vi "MOVE BIAS (M).vi"(0 "SweepQ In":refnum<queue>, 1 "x":dbl, 2 "return value":cluster{"x":dbl, "y":dbl}, 5 "ScanQ in":refnum<queue>, 7 "Boolean":bool, 11 "error in (no error)":errorcluster, 12 "y":dbl, 13 "Bias in":T1 {"Final Y (m)" format="%.3p"; "Final X (m)" format="%.3p"}) -> (3 "X (m)":sgl, 4 "SweepQ Out":refnum<queue>, 6 "ScanQ out":refnum<queue>, 14 "Y (m)":sgl, 15 "error out":errorcluster)   [LabVIEW 2025]
uses:
  STM-Auto-Project/QMH CTLS/Scan_Params (QMH).ctl
  LabVIEW VI's/Instrument VI's/Instrument Controls/Magnet Array.ctl
  Magnetic Drift Correction/Bias Cont QMH.ctl
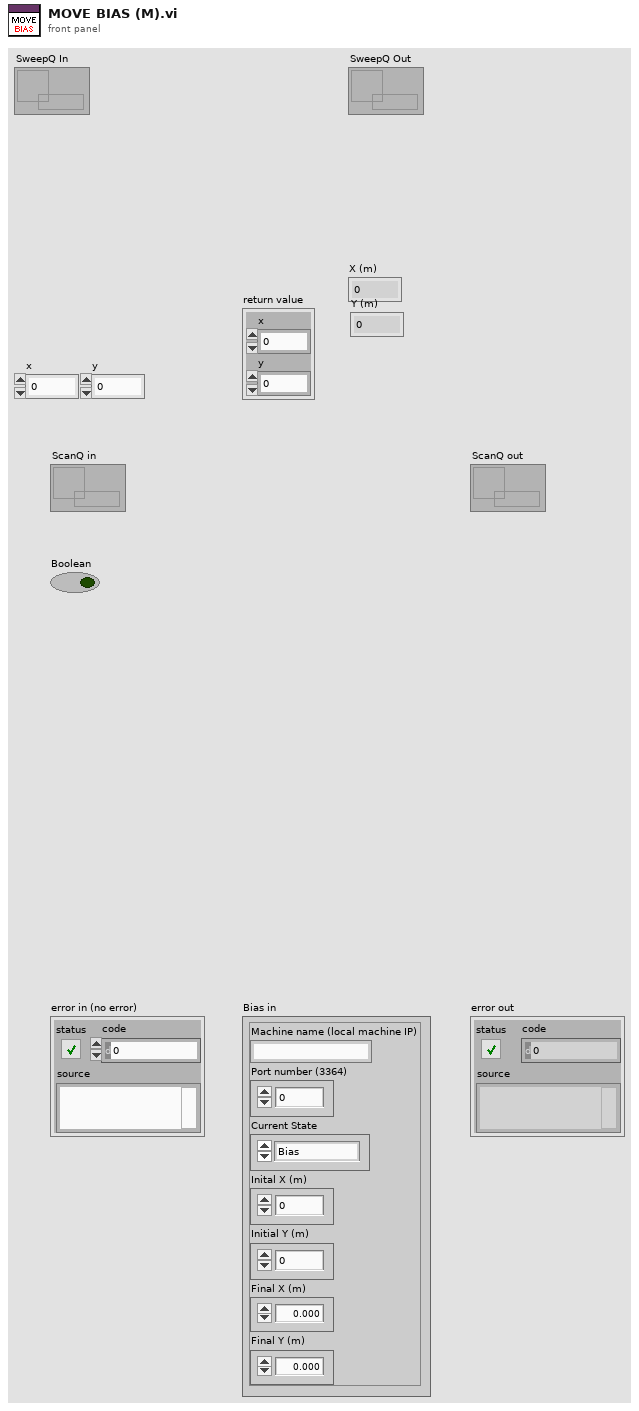
[diagram p1: front panel]
types:
  T1 = typedef "Bias Cont QMH.ctl" = cluster{"Machine name (local machine IP)":string, "Port number (3364)":u32, "Current State":enum16{"Bias", "Stop"}, "Inital X (m)":dbl, "Initial Y (m)":dbl, "Final X (m)":sgl, "Final Y (m)":sgl}
  T2 = enum16{"SET FIELD", "SWEEP IDLE", "NEXT FIELD", "SWEEP DONE"}
  T3 = typedef "Magnet Array.ctl" = cluster{"Sweep States":enum16{"SET FIELD", "SWEEP IDLE", "NEXT FIELD", "SWEEP DONE"}, "VISA Connection":refnum<visa-resource-name>, "Fields(T)":dbl[]}
  T4 = enum16{"1. BIAS", "2. INIT_SCAN", "3. SCAN_IDLE", "4. INTER_SCAN", "5. NEW_COORDS_&_FRAME", "6. FINAL_SCAN", "7. POLL BIAS ", "8. Z-CONT.", "9. STOP"}
  T5 = typedef "Scan_Params (QMH).ctl" = cluster{"Setpoint (I)":dbl[], "Bias (V)":dbl[], "Number of scans":u8, "Port number (3364)":u32, "Avoid zero threshold (V)":dbl, "Current State":enum16{"1. BIAS", "2. INIT_SCAN", "3. SCAN_IDLE", "4. INTER_SCAN", "5. NEW_COORDS_&_FRAME", "6. FINAL_SCAN", "7. POLL BIAS ", "8. Z-CONT.", "9. STOP"}}
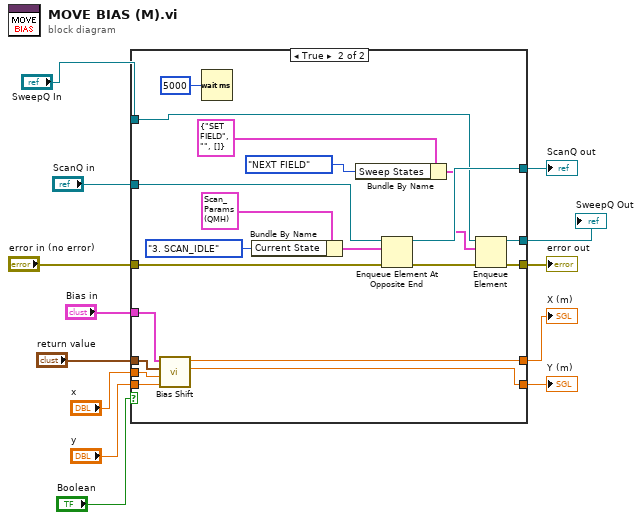
[diagram p0: block diagram]
diagram:
  n1 = case shown="True" "Boolean" {
    tunnel: "return value" -> [_ w30]
    tunnel: "ScanQ in" -> [w18 w34]
    tunnel: [w18 w35] -> w10
    tunnel: [w17 w36] -> w11
    tunnel: "error in (no error)" -> [w17 w32]
    tunnel: [w14 w37] -> w2
    tunnel: [w16 w29] -> w6
    tunnel: "Bias in" -> [_ w28]
    tunnel: [w15 w26] -> w5
    tunnel: "x" -> [w16 w25]
    tunnel: "y" -> [w15 w24]
    tunnel: "SweepQ In" -> [w14 w20]
    frame False {
    }
    frame True {
      n2 = call "Bias Shift.vi"("y"=w24, "x"=w25, "Translation (m)"=w30, "Bias Controller"=w28) -> ("Y (m)"=w26:sgl, "X (m)"=w29:sgl)  [unwired: 6 in]
      n3 = Wait (ms)(milliseconds to wait=u32 5000) -> ()  [unwired: 1 out]
      n4 = Bundle By Name(cluster=T5 {"Setpoint (I)"=[], "Bias (V)"=[], "Number of scans"=1, "Port number (3364)"=3364, "Avoid zero threshold (V)"=0.004999999888241291, "Current State"=enum."1. BIAS"} ("element"), "Current State"=T4."3. SCAN_IDLE") -> (w27:T5)
      n5 = Bundle By Name(cluster=T3 {"Sweep States"=enum."SET FIELD", "VISA Connection"="", "Fields(T)"=[]} ("element"), "Sweep States"=T2."NEXT FIELD") -> (w19:T3)
      n6 = Enqueue Element At Opposite End(queue=w34, element=w27, error in (no error)=w32) -> (queue out=w35:refnum<queue>, error out=w31:errorcluster)  [unwired: 1 in, 1 out]
      n7 = Enqueue Element(queue=w20, element=w19, error in (no error)=w31) -> (queue out=w37:refnum<queue>, error out=w36:errorcluster)  [unwired: 1 in, 1 out]
    }
  }
  "error out" <- w11
  "ScanQ out" <- w10
  "X (m)" <- w6
  "Y (m)" <- w5
  "SweepQ Out" <- w2
